vi "Ouverture_Porte_Handler.vi"(8 "Error In":errorcluster caption="Entrée d'erreur", 11 "Donnees_Globales_IN":T1) -> (0 "Error Out":errorcluster, 3 "Donnees_Globale_Out":T1)   [LabVIEW 2019]
uses:
  Asc_State_Inputs.ctl
  Etat_Asc.ctl
  <vilib>/Utility/error.llb/Error Cluster From Error Code.vi
  <vilib>/rvi/errors/niLvFpgaAdjustHostInterfaceError.vi
  <vilib>/rvi/interface/nirviReadWriteControl/nirviReadWriteControl.xnode
  NiFpgaLv.dll
  <vilib>/rvi/interface/Simulation/niFpgaSimulationCallBeginRW.vi
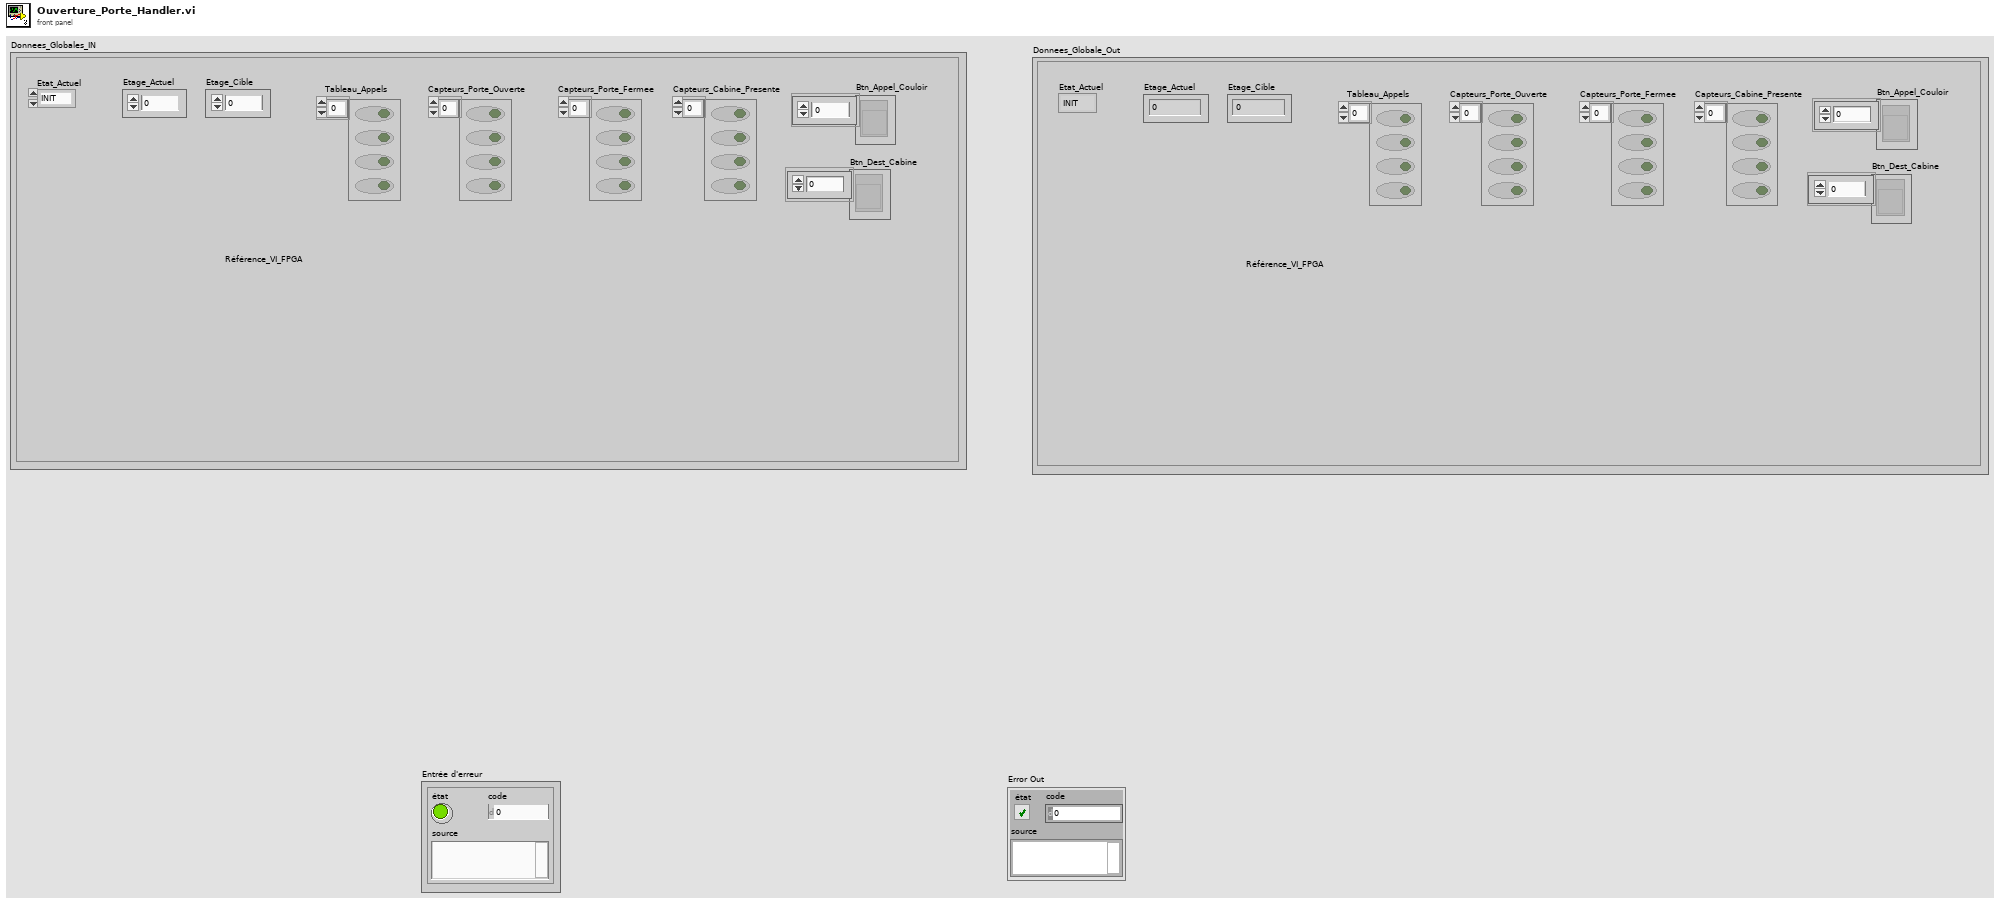
[diagram p1: front panel]
types:
  T1 = typedef "Asc_State_Inputs.ctl" = cluster{"Etage_Actuel":i32, "Etat_Actuel":T2, "Etage_Cible":i32, "Tableau_Appels":bool[], "Capteurs_Porte_Ouverte":bool[], "Capteurs_Porte_Fermee":bool[], "Capteurs_Cabine_Presente":bool[], "Btn_Appel_Couloir":refnum<vi>[], "Btn_Dest_Cabine":refnum<vi>[], "Référence_VI_FPGA":refnum<k20>}
  T2 = typedef "Etat_Asc.ctl" = enum16{"INIT", "REPOS", "DEPLACEMENT", "OUVERTURE_PORTE", "ATTENTE_TEMPO", "FERMETURE_PORTE", "ARRET_URGENCE"}
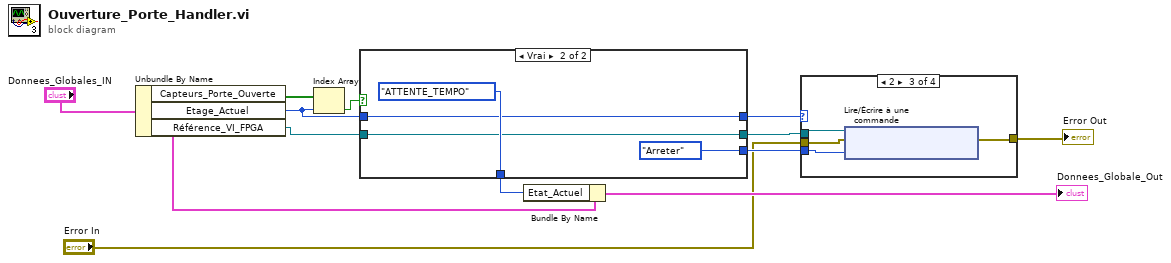
[diagram p0: block diagram]
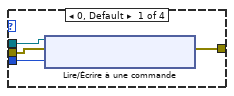
[diagram p2: hidden frame]
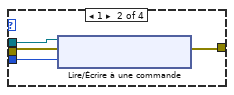
[diagram p3: hidden frame]
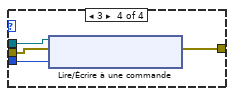
[diagram p4: hidden frame]
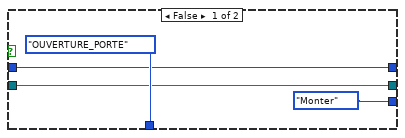
[diagram p5: hidden frame]
diagram:
  n1 = Unbundle By Name("Donnees_Globales_IN") -> ("Capteurs_Porte_Ouverte"=w12:bool[], "Etage_Actuel"=w7:i32, "Référence_VI_FPGA"=w8:refnum<k20>)
  n2 = Index Array(array=w12, index=w7) -> (element=w11:bool)
  n3 = case shown="Vrai" w11 {
    tunnel: [Etat_Asc."OUVERTURE_PORTE" ("Etat_Actuel") Etat_Asc."ATTENTE_TEMPO" ("Etat_Actuel")] -> w9
    tunnel: [w15 w19] -> w5
    tunnel: w8 -> [w15 w19]
    tunnel: w7 -> [w14 w18]
    tunnel: [w14 w18] -> w6
    tunnel: [enum16{"Monter", "Descendre", "Arreter"}."Monter" ("CMD_Moteur_Porte_1") enum16{"Monter", "Descendre", "Arreter"}."Arreter" ("CMD_Moteur_Porte_1")] -> w4
    frame False {
    }
    frame True {
    }
  }
  n4 = Bundle By Name(cluster="Donnees_Globales_IN", "Etat_Actuel"=w9) -> (→"Donnees_Globale_Out":T1)
  n5 = case shown="2" w6 {
    tunnel: w5 -> [w23 w28 w31 w35]
    tunnel: w4 -> [w24 w26 w32 w36]
    tunnel: [w22 w27 w30 w34] -> w3
    tunnel: "Error In" -> [w21 w25 w29 w33]
    frame 0, Default {
      n6 = xnode "Lire/Écrire à une commande"("Référence de VI FPGA en entrée"=w23, "entrée d'erreur"=w21, "CMD_Moteur_Porte_RDC"=w24) -> ("sortie d'erreur"=w22:errorcluster)  [unwired: 1 out]
    }
    frame 1 {
      n7 = xnode "Lire/Écrire à une commande"("Référence de VI FPGA en entrée"=w28, "entrée d'erreur"=w25, "CMD_Moteur_Porte_1"=w26) -> ("sortie d'erreur"=w27:errorcluster)  [unwired: 1 out]
    }
    frame 2 {
      n8 = xnode "Lire/Écrire à une commande"("Référence de VI FPGA en entrée"=w31, "entrée d'erreur"=w29, "CMD_Moteur_Porte_2"=w32) -> ("sortie d'erreur"=w30:errorcluster)  [unwired: 1 out]
    }
    frame 3 {
      n9 = xnode "Lire/Écrire à une commande"("Référence de VI FPGA en entrée"=w35, "entrée d'erreur"=w33, "CMD_Moteur_Porte_3"=w36) -> ("sortie d'erreur"=w34:errorcluster)  [unwired: 1 out]
    }
  }
  "Error Out" <- w3
